vi "get and update stim ring entries (subVI).vi"(8 "error in (no error)":errorcluster, 10 "odor-manifold config":T1, 11 "stim config array refnum":refnum<vi>) -> (0 "error out":errorcluster, 3 "stim config array refnum out":refnum<vi>)   [LabVIEW 2021]
uses:
  type-defs/odor and manifold config cluster (type def).ctl
  type-defs/manifold configuration cluster array (type def).ctl
  type-defs/manifold configuration cluster (type def).ctl
  type-defs/manifold selection.ctl
  type-defs/single port single odor cluster.ctl
  type-defs/port number (type def).ctl
  type-defs/odor selection (type def).ctl
  type-defs/odor color (type def).ctl
  type-defs/odor description array (type def).ctl
  type-defs/odor info cluster (type def).ctl
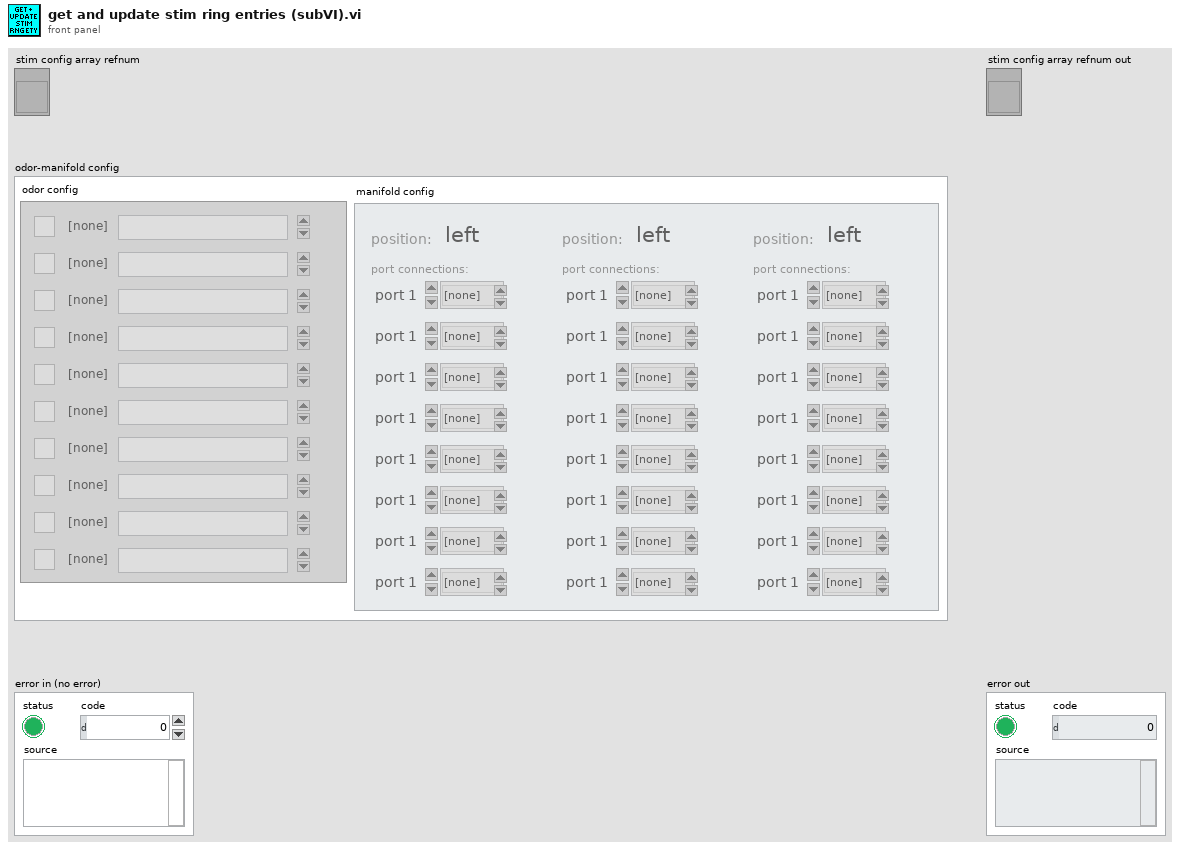
[diagram p1: front panel]
types:
  T1 = typedef "odor and manifold config cluster (type def).ctl" = cluster{"manifold config":T2, "odor config":T9}
  T2 = typedef "manifold configuration cluster array (type def).ctl" = T3[]
  T3 = typedef "manifold configuration cluster (type def).ctl" = cluster{"position:":T4, "port connections:":T5[]}
  T4 = typedef "manifold selection.ctl" = enum16{"left", "middle", "right"}
  T5 = typedef "single port single odor cluster.ctl" = cluster{"port number":T6, "connected odor":T7, "error":bool, "odor color":T8}
  T6 = typedef "port number (type def).ctl" = enum16{"port 1", "port 2", "port 3", "port 4", "port 5", "port 6", "port 7", "port 8"}
  T7 = typedef "odor selection (type def).ctl" = enum16{"[none]", "odor 1", "odor 2", "odor 3", "odor 4", "odor 5", "odor 6", "odor 7", "odor 8", "odor 9", "odor 10"}
  T8 = typedef "odor color (type def).ctl" = u16
  T9 = typedef "odor description array (type def).ctl" = T10[]
  T10 = typedef "odor info cluster (type def).ctl" = cluster{"odor channel":T7, "odor description":string, "odor color":T8, "odor channel active":bool}
  T11 = cluster{"stim. config line cluster":refnum<vi>, "description string":refnum<vi>, "duration, s numeric":refnum<vi>, "port-odor & color cluster []":refnum<vi>[], "port-odor ring []":refnum<vi>[], "odor color ring []":refnum<vi>[]}
  T12 = typedef "ragged ring entry 2D array cluster (typed def).ctl" = cluster{"StringAndValue[][]":T13[][], "Size[]":i32[]}
  T13 = typedef "ring string and value cluster (type def).ctl" = cluster{"String":string, "Value":u16}
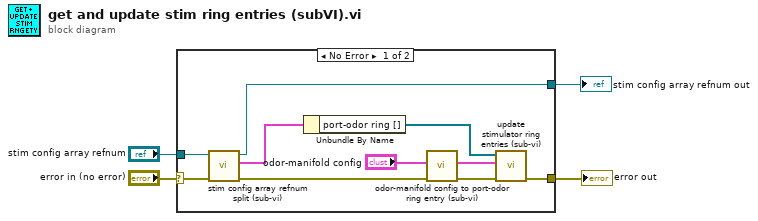
[diagram p0: block diagram]
diagram:
  n1 = case shown="No Error" "error in (no error)" {
    selector: "error in (no error)" -> [w8 w15]
    tunnel: "stim config array refnum" -> [w12 w16]
    tunnel: [w11 w15] -> w3
    tunnel: [w5 w16] -> w1
    frame No Error {
      n2 = call "stim config array refnum split (sub-vi).vi"("error in (no error)"=w8, "stim. config array refnum"=w12) -> ("error out"=w13:errorcluster, "element refnum cluster"=w6:T11, "stim. config array refnum out"=w5:refnum<vi>)  [unwired: 7 in]
      n3 = Unbundle By Name(w6) -> ("port-odor ring []"=w10:refnum<vi>[])
      n4 = call "odor-manifold config to port-odor ring entry (sub-vi).vi"("error in (no error)"=w13, "odor-manifold config"="odor-manifold config") -> ("error out"=w9:errorcluster, "ragged ring entry 2D array"=w7:T12)  [unwired: 8 in]
      n5 = call "update stimulator ring entries (sub-vi).vi"("error in (no error)"=w9, "ragged ring entry []"=w7, "port-odor ring refnum []"=w10) -> ("error out"=w11:errorcluster)  [unwired: 7 in, 1 out]
    }
    frame Error {
    }
  }
  "error out" <- w3
  "stim config array refnum out" <- w1
